vi "Config.vi"() -> ()   [LabVIEW 2020]
uses:
  Global_Variable/Global.vi
  Global_Variable/A180648.vi
  <vilib>/Utility/config.llb/NI_LVConfig.lvlib
  Libraries/S7/S7.lvlib
panel:
  in  "系数":bool
  in  "试验项目":T1
  in  "产品型号":string(combo)
  in  "删除":bool
  in  "确定":bool
  in  "添加":bool
  in  "退出":bool
  in  "更新":bool
  in  "选项卡控件":enum32{"产品参数", "系统参数"}(tab)
  in  "开启 3":string[][](table)=[["N"], ["N"], ["N"], ["mm"]]
  in  "开启 2":string[][](table)=[["N"], ["N"], ["N"], ["mm"]]
  in  "开启":string[][](table)=[["N"], ["N"], ["N"], ["mm"]]
  in  "工位坐标轴参数":string[][](table)=[["°"], ["N"], ["°"], ["N"], ["mm"], ["N"], ["mm"], ["N"]]
  in  "结果判定参数":string[][](table)=[["N"], ["N"], ["N"], ["mm"]]
  in  "系统参数设置":string[][](table)=[[""], ["mm"], ["V"], [""]]
  # "调节机构检测"
types:
  T1 = cluster{"锁紧力":bool, "开启力":bool, "推拉力":bool, "保持力":bool, "锁紧/开启":bool}
  T2 = enum8{"Enabled", "Disabled", "Disabled and Grayed Out"}
  T3 = typedef "NI_LVConfig.lvlib/Config Data RefNum.ctl" = refnum<k1>
  T4 = cluster{"[0]":cluster{string, dbl, dbl}, "[1]":cluster{string, dbl, dbl}}
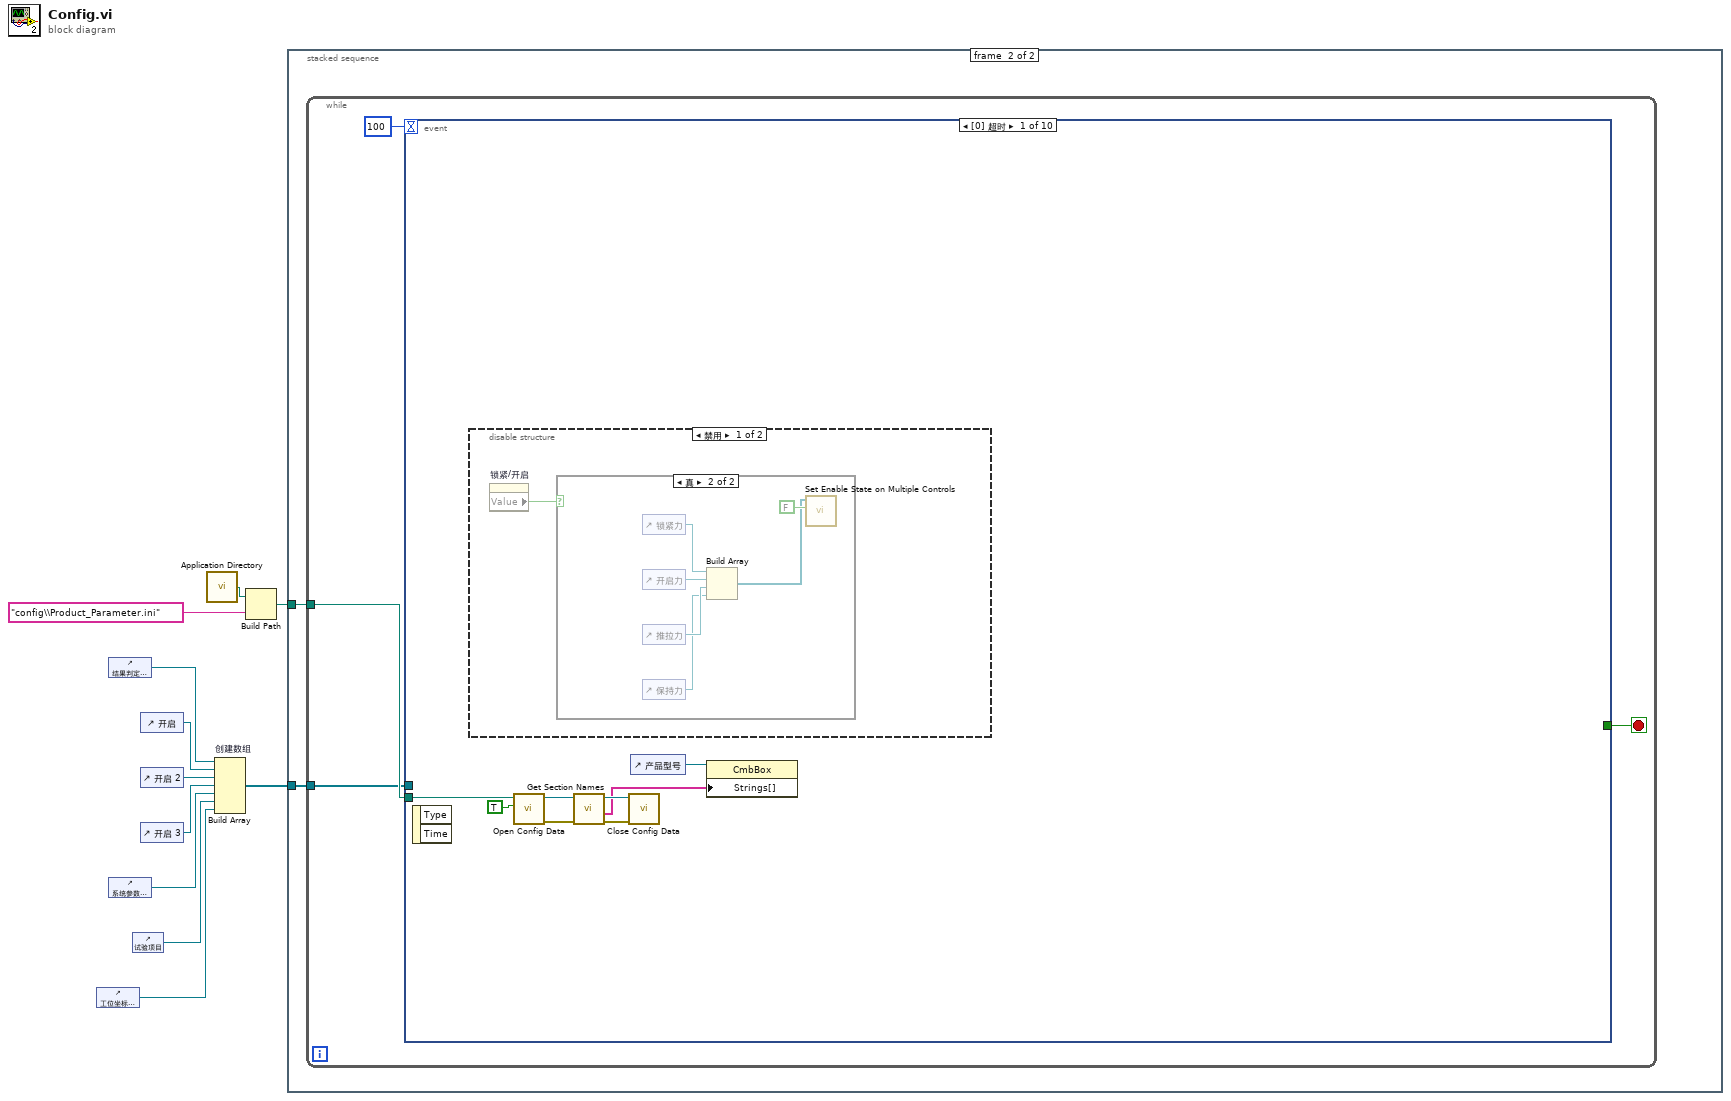
[diagram p0: block diagram]
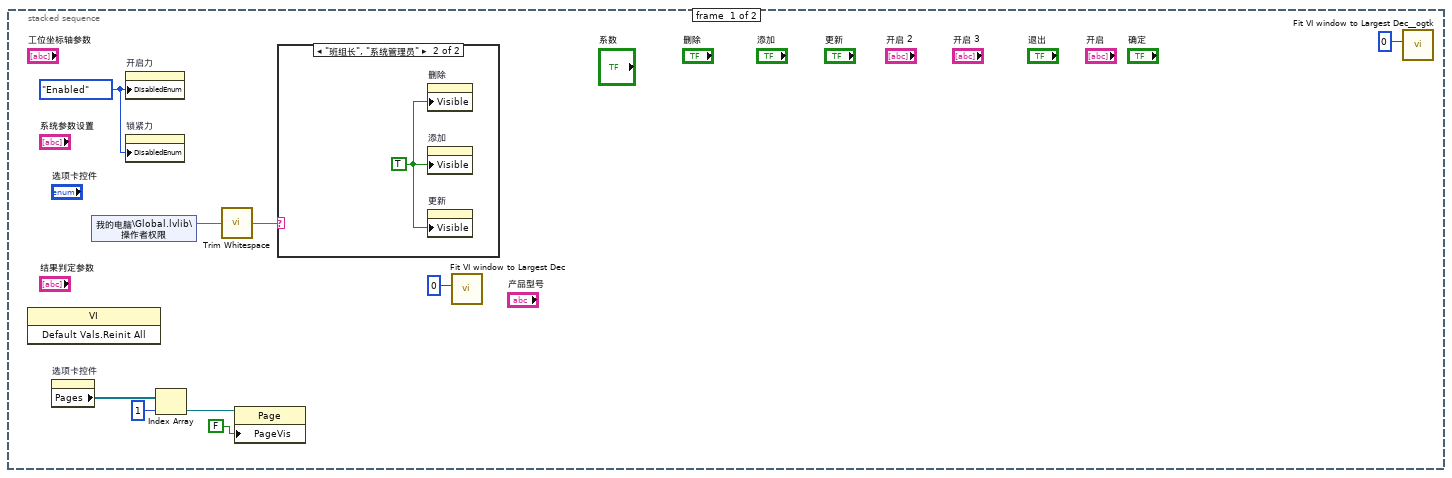
[diagram p2: hidden frame]
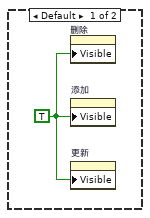
[diagram p3: hidden frame]
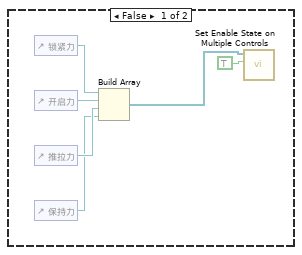
[diagram p4: hidden frame]
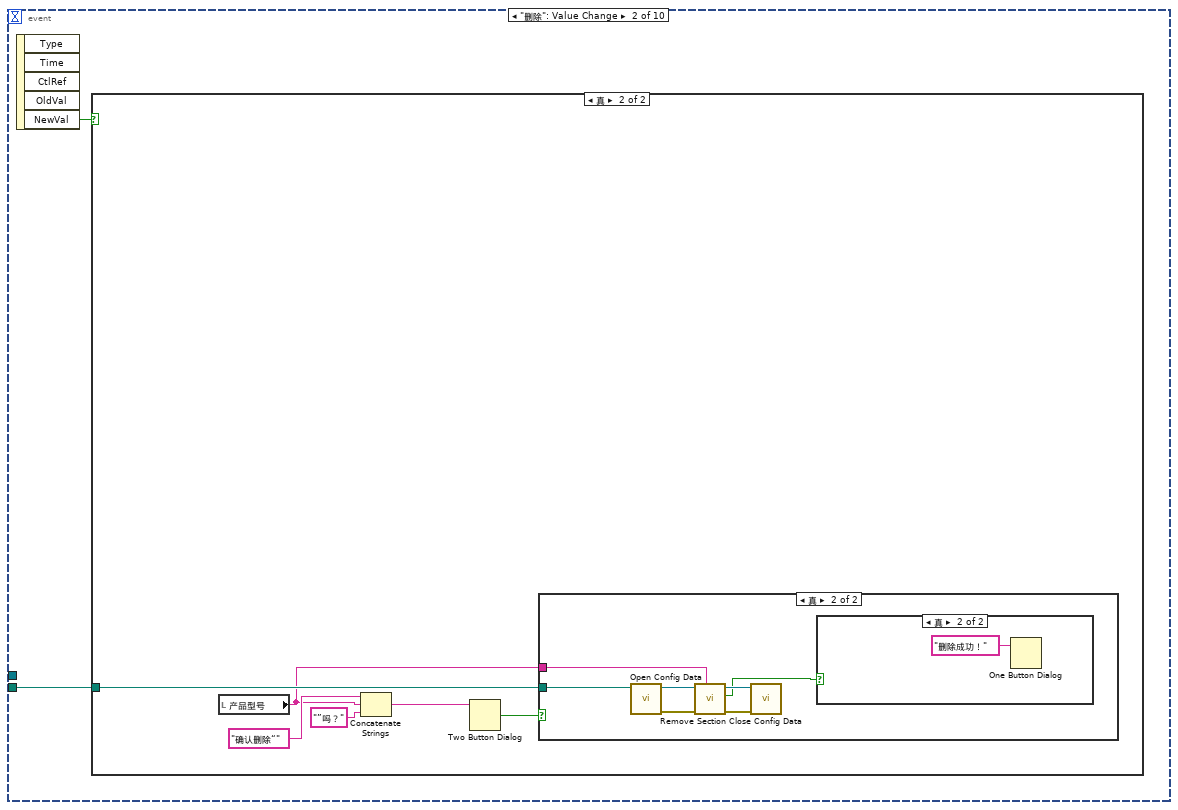
[diagram p6: hidden frame]
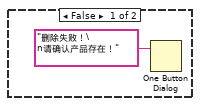
[diagram p9: hidden frame]
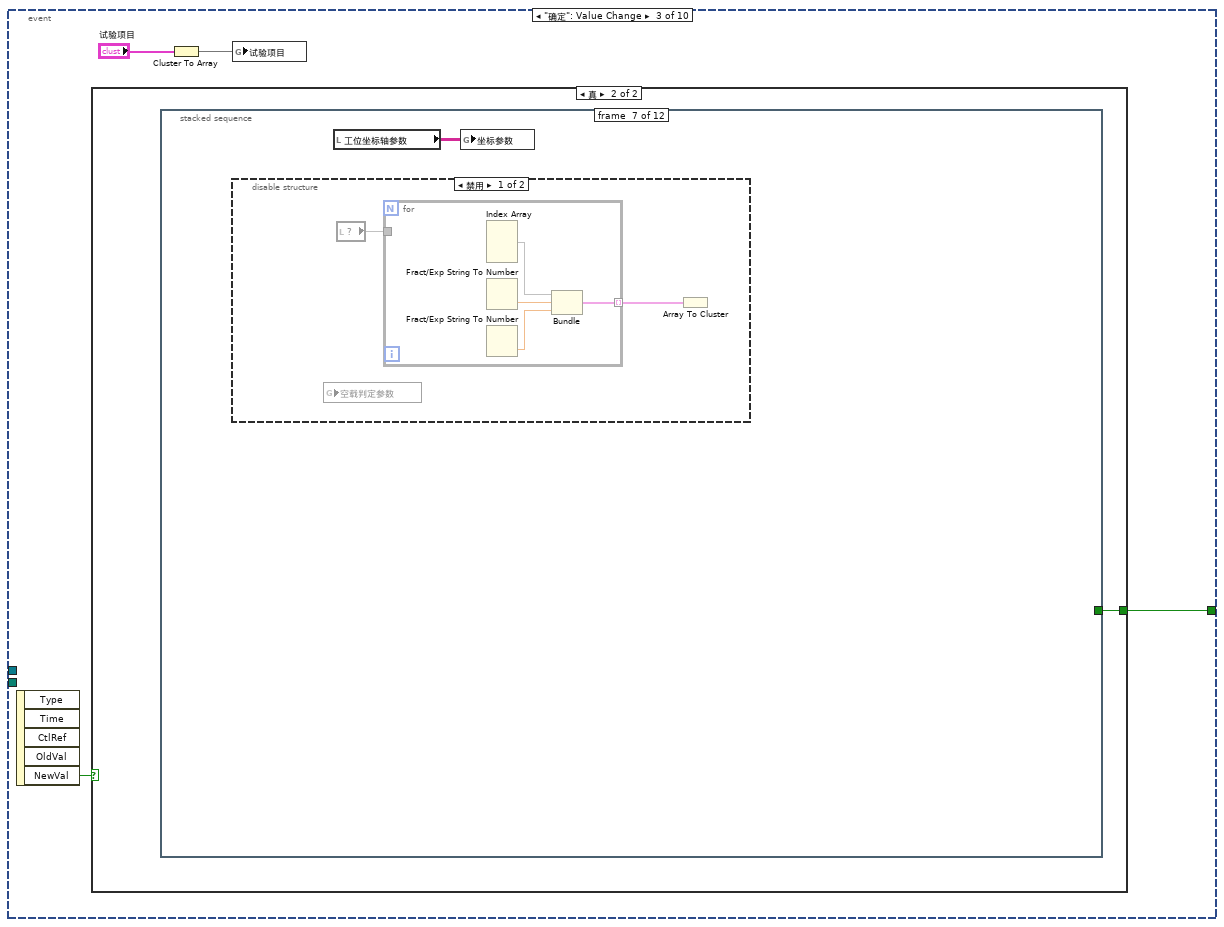
[diagram p10: hidden frame]
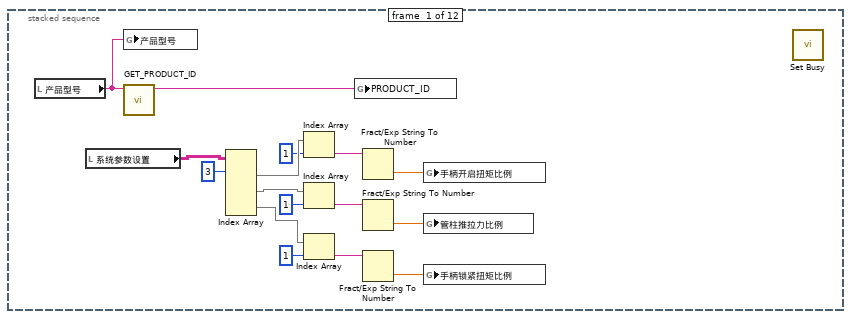
[diagram p12: hidden frame]
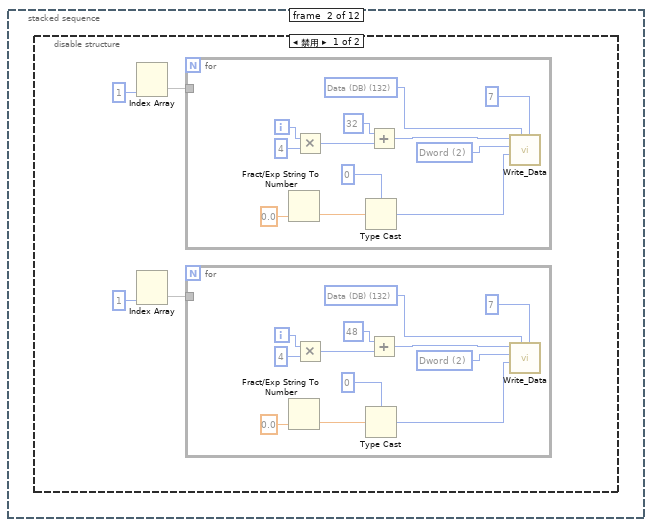
[diagram p13: hidden frame]
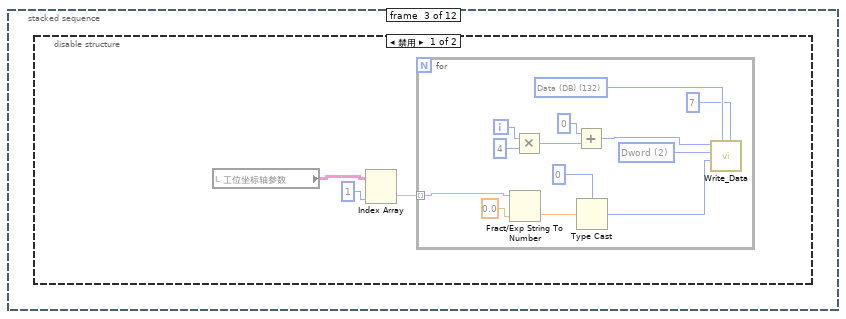
[diagram p15: hidden frame]
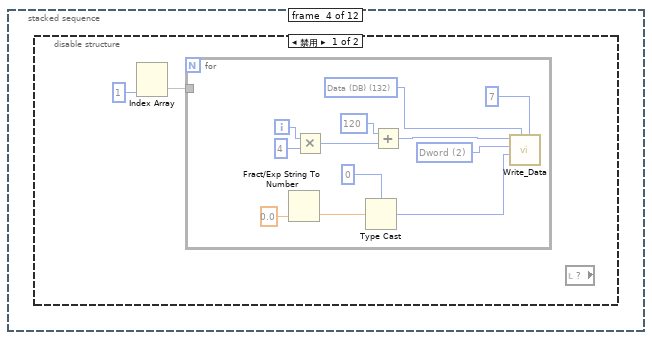
[diagram p17: hidden frame]
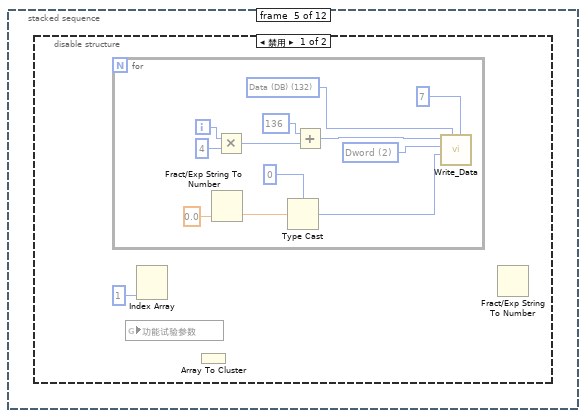
[diagram p19: hidden frame]
diagram:
  n1 = control-ref of="工位坐标轴参数"() -> (w1:refnum<vi>)
  n2 = control-ref of="结果判定参数"() -> (w7:refnum<vi>)
  n3 = control-ref of="系统参数设置"() -> (w8:refnum<vi>)
  n4 = control-ref of="试验项目"() -> (w2:refnum<vi>)
  n5 = control-ref of="开启"() -> (w5:refnum<vi>)
  n6 = control-ref of="开启 2"() -> (w4:refnum<vi>)
  n7 = control-ref of="开启 3"() -> (w3:refnum<vi>)
  n8 = call <vilib>:"Application Directory.vi"() -> ("Application Directory"=w10:path)
  n9 = Build Array "创建数组"(w7, w5, w4, w3, w8, w2, w1) -> (w11:refnum<vi>[])
  n10 = Build Path(base path=w10, name or relative path="config\\Product_Parameter.ini" ("名称或相对路径")) -> (appended path=w9:path)
  n11 = stacked-sequence {
    tunnel: w11 -> [_ w23]
    tunnel: w9 -> [_ w24]
    frame #0 {
      w16 = T2."Enabled" ("禁用")
      n12 = invoke class="VI" method="Default Vals.Reinit All"() -> ()  [unwired: 3 in, 3 out]
      n13 = property on="选项卡控件" class="TabCtl (严格)"() -> ("Pages"=w14:refnum<vi>[])  [unwired: 2 in, 2 out]
      n14 = shared-variable "我的电脑\\Global.lvlib\\操作者权限"() -> (w20:string)  [unwired: 1 in, 1 out]
      n15 = property on="开启力" class="Bool (严格)"("DisabledEnum"=w16) -> ()  [unwired: 2 in, 2 out]
      n16 = property on="锁紧力" class="Bool (严格)"("DisabledEnum"=w16) -> ()  [unwired: 2 in, 2 out]
      n17 = Index Array(array=w14, index=1 ("索引")) -> (element=w15:refnum<vi>)
      n18 = call <vilib>:"Trim Whitespace.vi"("string"=w20) -> ("trimmed string"=w19:string)  [unwired: 1 in]
      n19 = property class="Page"(reference=w15, "PageVis"=FALSE ("选项卡可见")) -> ()  [unwired: 1 in, 2 out]
      n20 = case shown="\"班组长\", \"系统管理员\"" w19 {
        frame Default {
          w21 = TRUE ("可见")
          n21 = property on="删除" class="Bool (严格)"("Visible"=w21) -> ()  [unwired: 2 in, 2 out]
          n22 = property on="添加" class="Bool (严格)"("Visible"=w21) -> ()  [unwired: 2 in, 2 out]
          n23 = property on="更新" class="Bool (严格)"("Visible"=w21) -> ()  [unwired: 2 in, 2 out]
        }
        frame "班组长", "系统管理员" {
          w22 = TRUE ("可见")
          n24 = property on="删除" class="Bool (严格)"("Visible"=w22) -> ()  [unwired: 2 in, 2 out]
          n25 = property on="添加" class="Bool (严格)"("Visible"=w22) -> ()  [unwired: 2 in, 2 out]
          n26 = property on="更新" class="Bool (严格)"("Visible"=w22) -> ()  [unwired: 2 in, 2 out]
        }
      }
      n27 = call "Fit VI window to Largest Dec.vi"("border spacing (2 px)"=0) -> ()  [unwired: 5 in, 2 out]
      n28 = call <userlib>:"Fit VI window to Largest Dec__ogtk.vi"("border spacing (2 px)"=0) -> ()  [unwired: 5 in, 2 out]
    }
    frame #1 {
      n29 = while {
        tunnel: w24 -> [w28]
        tunnel: w23 -> [w25]
        stop <- w27 stop-if-true
        n30 = event shown="[0] 超时" {
          selector: _ -> [_ _ _ _ _ _ _ _ _ _]
          dyn-events: _ -> [_ _ _ _ _ _ _ _ _ _]
          timeout: 100 -> [_ _ _ _ _ _ _ _ _ _]
          tunnel: w28 -> [w31 w51 _ w245 w273 _ w296 _ _ _]
          tunnel: [_ _ w69 _ _ TRUE _ _ _ TRUE] -> w27
          tunnel: w25 -> [_ _ _ w243 w271 _ w294 _ _ _]
          event Timeout {
            n31 = event-data() -> ()  [unwired: 1 in, 2 out]
            n32 = disable-structure shown="禁用" {
              frame Disabled {
                n33 = property on="锁紧/开启" class="Bool (严格)"() -> ("Value"=w37:bool)  [unwired: 2 in, 2 out]
                n34 = case shown="真" w37 {
                  frame False {
                    n35 = control-ref of="锁紧力"() -> (w42:refnum<vi>)
                    n36 = control-ref of="开启力"() -> (w41:refnum<vi>)
                    n37 = control-ref of="推拉力"() -> (w40:refnum<vi>)
                    n38 = control-ref of="保持力"() -> (w39:refnum<vi>)
                    n39 = Build Array(w42, w41, w40, w39) -> (w38:refnum<vi>[])
                    n40 = call "Set Enable State on Multiple Controls.vi"("启用？"=TRUE, "控件"=w38) -> ()  [unwired: 10 in]
                  }
                  frame True {
                    n41 = control-ref of="锁紧力"() -> (w48:refnum<vi>)
                    n42 = control-ref of="开启力"() -> (w47:refnum<vi>)
                    n43 = control-ref of="推拉力"() -> (w46:refnum<vi>)
                    n44 = control-ref of="保持力"() -> (w45:refnum<vi>)
                    n45 = Build Array(w48, w47, w46, w45) -> (w44:refnum<vi>[])
                    n46 = call "Set Enable State on Multiple Controls.vi"("启用？"=FALSE, "控件"=w44) -> ()  [unwired: 10 in]
                  }
                }
              }
              frame Enabled {
              }
            }
            n47 = call <vilib>:"Open Config Data.vi"("create file if necessary (T)"=TRUE, "configuration file path"=w31) -> ("error out"=w33:errorcluster, "refnum"=w32:T3)  [unwired: 7 in, 1 out]
            n48 = call <vilib>:"Get Section Names.vi"("error in (no error)"=w33, "refnum"=w32) -> ("error out"=w35:errorcluster, "section names"=w29:string[], "refnum out"=w34:T3)  [unwired: 7 in]
            n49 = call <vilib>:"Close Config Data.vi"("error in (no error)"=w35, "refnum"=w34) -> ()  [unwired: 8 in, 2 out]
            n50 = control-ref of="产品型号"() -> (w30:refnum<vi>)
            n51 = property on="属性节点" class="CmbBox"(reference=w30, "Strings[]"=w29) -> ()  [unwired: 1 in, 2 out]
          }
          event "删除": Value Change {
            n52 = event-data() -> ("NewVal"=w50:bool)  [unwired: 1 in, 4 out]
            n53 = case shown="真" w50 {
              tunnel: w51 -> [_ w53]
              frame False {
              }
              frame True {
                n54 = local read "产品型号"() -> (w52:string)
                n55 = Concatenate Strings("确认删除“", w52, "”吗？") -> (w55:string)
                n56 = Two Button Dialog(message=w55) -> (T button?=w54:bool)  [unwired: 2 in]
                n57 = case shown="真" w54 {
                  tunnel: w53 -> [_ w59]
                  tunnel: w52 -> [_ w58]
                  frame False {
                  }
                  frame True {
                    n58 = call <vilib>:"Open Config Data.vi"("configuration file path"=w59) -> ("error out"=w61:errorcluster, "refnum"=w64:T3)  [unwired: 8 in, 1 out]
                    n59 = call <vilib>:"Remove Section.vi"("section"=w58, "error in (no error)"=w61, "refnum"=w64) -> ("error out"=w63:errorcluster, "section exists?"=w60:bool, "refnum out"=w62:T3)  [unwired: 6 in]
                    n60 = call <vilib>:"Close Config Data.vi"("error in (no error)"=w63, "refnum"=w62) -> ()  [unwired: 8 in, 2 out]
                    n61 = case shown="真" w60 {
                      frame False {
                        n62 = One Button Dialog(message="删除失败！\n请确认产品存在！" ("消息")) -> ()  [unwired: 1 in, 1 out]
                      }
                      frame True {
                        n63 = One Button Dialog(message="删除成功！" ("消息")) -> ()  [unwired: 1 in, 1 out]
                      }
                    }
                  }
                }
              }
            }
          }
          event "确定": Value Change {
            n64 = event-data() -> ("NewVal"=w70:bool)  [unwired: 1 in, 4 out]
            n65 = case shown="真" w70 {
              tunnel: [_ w71] -> w69
              frame False {
              }
              frame True {
                n66 = stacked-sequence {
                  tunnel: [_ _ _ _ _ _ _ _ _ _ _ TRUE] -> w71
                  frame #0 {
                    n67 = local read "产品型号"() -> (w87:string)
                    n68 = local read "系统参数设置"() -> (w85:string[][])
                    n69 = global write "Global.vi" "产品型号"(w87) -> ()
                    n70 = call "GET_PRODUCT_ID.vi"("PRODFUCT_NAME"=w87) -> ("PRODUCT_ID"=w86:string)  [unwired: 10 in]
                    n71 = Index Array(array=w85, index (row) #1=3 ("索引 (行)")) -> (element #1=w83:string[], element #2=w77:string[], element #3=w74:string[])  [unwired: 5 in]
                    n72 = Index Array(array=w83, index=1 ("索引")) -> (element=w81:string)
                    n73 = Index Array(array=w77, index=1 ("索引")) -> (element=w79:string)
                    n74 = Index Array(array=w74, index=1 ("索引")) -> (element=w73:string)
                    n75 = global write "追溯Global.vi" "PRODUCT_ID"(w86) -> ()
                    n76 = Fract/Exp String To Number(string=w81) -> (number=w80:dbl)  [unwired: 3 in, 1 out]
                    n77 = Fract/Exp String To Number(string=w79) -> (number=w76:dbl)  [unwired: 3 in, 1 out]
                    n78 = Fract/Exp String To Number(string=w73) -> (number=w72:dbl)  [unwired: 3 in, 1 out]
                    n79 = global write "A180648.vi" "手柄开启扭矩比例"(w80) -> ()
                    n80 = global write "A180648.vi" "管柱推拉力比例"(w76) -> ()
                    n81 = global write "A180648.vi" "手柄锁紧扭矩比例"(w72) -> ()
                    n82 = call <vilib>:"Set Busy.vi"() -> ()  [unwired: 10 in, 2 out]
                  }
                  frame #1 {
                    n83 = disable-structure shown="禁用" {
                      frame Disabled {
                        n84 = Index Array(index (col)=1 ("禁用的索引 (列)")) -> (element=w91)  [unwired: 2 in]
                        n85 = Index Array(index (col)=1 ("禁用的索引 (列)")) -> (element=w88)  [unwired: 2 in]
                        n86 = for {
                          tunnel: w91 -> [_]
                          i -> [w106]
                          w113 = u16 2 items=["byte", "word", "Dword"] ("数据类型")
                          w115 = u8 132 items=["I/O (P)"=128, "Input (I)"=129, "Output (Q)"=130, "Bit Memory (M)"=131, "Data (DB)"=132, "Instance Data (DI)"=133, "Local Data (L)"=134, "Predecessor Local Data (VL)"=135] ("寄存器类型")
                          n87 = Fract/Exp String To Number(default (0 dbl)=sgl 0.0) -> (number=w110:sgl)  [unwired: 3 in, 1 out]
                          n88 = Multiply(x=w106, y=4) -> (x*y=w107:i32)
                          n89 = Type Cast(type=u32 0 ("写入地址"), x=w110) -> (*(type *) &x=w109:u32)
                          n90 = Add(x=u32 32 ("写入地址"), y=w107) -> (x+y=w104:u32)
                          n91 = call "Write_Data.vi"("DB #"=u16 7, "寄存器类型"=w115, "写入数据"=w109, "数据类型"=w113, "写入地址"=w104) -> ()  [unwired: 4 in, 3 out]
                        }
                        n92 = for {
                          tunnel: w88 -> [_]
                          i -> [w94]
                          w101 = u16 2 items=["byte", "word", "Dword"] ("数据类型")
                          w103 = u8 132 items=["I/O (P)"=128, "Input (I)"=129, "Output (Q)"=130, "Bit Memory (M)"=131, "Data (DB)"=132, "Instance Data (DI)"=133, "Local Data (L)"=134, "Predecessor Local Data (VL)"=135] ("寄存器类型")
                          n93 = Fract/Exp String To Number(default (0 dbl)=sgl 0.0) -> (number=w98:sgl)  [unwired: 3 in, 1 out]
                          n94 = Multiply(x=w94, y=4) -> (x*y=w95:i32)
                          n95 = Type Cast(type=u32 0 ("写入地址"), x=w98) -> (*(type *) &x=w97:u32)
                          n96 = Add(x=u32 48 ("写入地址"), y=w95) -> (x+y=w92:u32)
                          n97 = call "Write_Data.vi"("DB #"=u16 7, "寄存器类型"=w103, "写入数据"=w97, "数据类型"=w101, "写入地址"=w92) -> ()  [unwired: 4 in, 3 out]
                        }
                      }
                      frame Enabled {
                      }
                    }
                  }
                  frame #2 {
                    n98 = disable-structure shown="禁用" {
                      frame Disabled {
                        n99 = local read "工位坐标轴参数"() -> (w118:string[][])
                        n100 = Index Array(array=w118, index (col)=1 ("禁用的索引 (列)")) -> (element=w117:string[])  [unwired: 1 in]
                        n101 = for {
                          tunnel: w117 -> [w127] mode=indexing
                          i -> [w121]
                          w129 = u16 2 items=["byte", "word", "Dword"] ("数据类型")
                          w131 = u8 132 items=["I/O (P)"=128, "Input (I)"=129, "Output (Q)"=130, "Bit Memory (M)"=131, "Data (DB)"=132, "Instance Data (DI)"=133, "Local Data (L)"=134, "Predecessor Local Data (VL)"=135] ("寄存器类型")
                          n102 = Fract/Exp String To Number(string=w127, default (0 dbl)=sgl 0.0) -> (number=w125:sgl)  [unwired: 2 in, 1 out]
                          n103 = Multiply(x=w121, y=4) -> (x*y=w122:i32)
                          n104 = Add(x=u32 0 ("写入地址"), y=w122) -> (x+y=w119:u32)
                          n105 = Type Cast(type=u32 0 ("写入地址"), x=w125) -> (*(type *) &x=w124:u32)
                          n106 = call "Write_Data.vi"("DB #"=u16 7, "寄存器类型"=w131, "写入数据"=w124, "数据类型"=w129, "写入地址"=w119) -> ()  [unwired: 4 in, 3 out]
                        }
                      }
                      frame Enabled {
                      }
                    }
                  }
                  frame #3 {
                    n107 = disable-structure shown="禁用" {
                      frame Disabled {
                        n108 = Index Array(index (col)=1 ("禁用的索引 (列)")) -> (element=w133)  [unwired: 2 in]
                        n109 = for {
                          tunnel: w133 -> [_]
                          i -> [w136]
                          w143 = u16 2 items=["byte", "word", "Dword"] ("数据类型")
                          w145 = u8 132 items=["I/O (P)"=128, "Input (I)"=129, "Output (Q)"=130, "Bit Memory (M)"=131, "Data (DB)"=132, "Instance Data (DI)"=133, "Local Data (L)"=134, "Predecessor Local Data (VL)"=135] ("寄存器类型")
                          n110 = Fract/Exp String To Number(default (0 dbl)=sgl 0.0) -> (number=w140:sgl)  [unwired: 3 in, 1 out]
                          n111 = Multiply(x=w136, y=4) -> (x*y=w137:i32)
                          n112 = Type Cast(type=u32 0 ("写入地址"), x=w140) -> (*(type *) &x=w139:u32)
                          n113 = Add(x=u32 120 ("写入地址"), y=w137) -> (x+y=w134:u32)
                          n114 = call "Write_Data.vi"("DB #"=u16 7, "寄存器类型"=w145, "写入数据"=w139, "数据类型"=w143, "写入地址"=w134) -> ()  [unwired: 4 in, 3 out]
                        }
                        n115 = local read item#-1() -> ()  [unwired: 1 out]
                      }
                      frame Enabled {
                      }
                    }
                  }
                  frame #4 {
                    n116 = disable-structure shown="禁用" {
                      frame Disabled {
                        n117 = for {
                          i -> [w149]
                          w156 = u16 2 items=["byte", "word", "Dword"] ("数据类型")
                          w158 = u8 132 items=["I/O (P)"=128, "Input (I)"=129, "Output (Q)"=130, "Bit Memory (M)"=131, "Data (DB)"=132, "Instance Data (DI)"=133, "Local Data (L)"=134, "Predecessor Local Data (VL)"=135] ("寄存器类型")
                          n118 = Fract/Exp String To Number(default (0 dbl)=sgl 0.0) -> (number=w153:sgl)  [unwired: 3 in, 1 out]
                          n119 = Multiply(x=w149, y=4) -> (x*y=w150:i32)
                          n120 = Type Cast(type=u32 0 ("写入地址"), x=w153) -> (*(type *) &x=w152:u32)
                          n121 = Add(x=u32 136 ("写入地址"), y=w150) -> (x+y=w147:u32)
                          n122 = call "Write_Data.vi"("DB #"=u16 7, "寄存器类型"=w158, "写入数据"=w152, "数据类型"=w156, "写入地址"=w147) -> ()  [unwired: 4 in, 3 out]
                        }
                        n123 = global read "A180648.vi" "功能试验参数"() -> ()  [unwired: 1 in]
                        n124 = Index Array(index (col)=1 ("禁用的索引 (列)")) -> ()  [unwired: 2 in, 1 out]
                        n125 = Array To Cluster() -> ()  [unwired: 1 in, 1 out]
                        n126 = Fract/Exp String To Number() -> ()  [unwired: 4 in, 2 out]
                      }
                      frame Enabled {
                      }
                    }
                  }
                  frame #5 {
                    n127 = disable-structure shown="禁用" {
                      frame Disabled {
                        n128 = for {
                          i -> [w162]
                          w169 = u16 2 items=["byte", "word", "Dword"] ("数据类型")
                          w171 = u8 132 items=["I/O (P)"=128, "Input (I)"=129, "Output (Q)"=130, "Bit Memory (M)"=131, "Data (DB)"=132, "Instance Data (DI)"=133, "Local Data (L)"=134, "Predecessor Local Data (VL)"=135] ("寄存器类型")
                          n129 = Fract/Exp String To Number(default (0 dbl)=sgl 0.0) -> (number=w166:sgl)  [unwired: 3 in, 1 out]
                          n130 = Multiply(x=w162, y=4) -> (x*y=w163:i32)
                          n131 = Type Cast(type=u32 0 ("写入地址"), x=w166) -> (*(type *) &x=w165:u32)
                          n132 = Add(x=u32 168 ("写入地址"), y=w163) -> (x+y=w160:u32)
                          n133 = call "Write_Data.vi"("DB #"=u16 7, "寄存器类型"=w171, "写入数据"=w165, "数据类型"=w169, "写入地址"=w160) -> ()  [unwired: 4 in, 3 out]
                        }
                        n134 = global read "A180648.vi" "逆向空载试验参数"() -> ()  [unwired: 1 in]
                        n135 = Index Array(index (col)=1 ("禁用的索引 (列)")) -> ()  [unwired: 2 in, 1 out]
                        n136 = Fract/Exp String To Number() -> ()  [unwired: 4 in, 2 out]
                        n137 = Array To Cluster() -> ()  [unwired: 1 in, 1 out]
                      }
                      frame Enabled {
                      }
                    }
                  }
                  frame #6 {
                    n138 = disable-structure shown="禁用" {
                      frame Disabled {
                        n139 = global read "判定参数.vi" "空载判定参数"() -> ()  [unwired: 1 in]
                        n140 = local read item#-1() -> (w174)
                        n141 = for {
                          tunnel: w174 -> [_]
                          tunnel: [w176] -> w173 mode=indexing
                          n142 = Index Array() -> (element #1=w175)  [unwired: 4 in, 2 out]
                          n143 = Fract/Exp String To Number() -> (number=w178:dbl)  [unwired: 4 in, 1 out]
                          n144 = Fract/Exp String To Number() -> (number=w177:dbl)  [unwired: 4 in, 1 out]
                          n145 = Bundle(w175, w178, w177) -> (w176:cluster{void, dbl, dbl})  [unwired: 1 in]
                        }
                        n146 = Array To Cluster(array=w173) -> ()  [unwired: 1 out]
                      }
                      frame Enabled {
                      }
                    }
                    n147 = local read "工位坐标轴参数"() -> (w172:string[][])
                    n148 = global write "A180648.vi" "坐标参数"(w172) -> ()
                  }
                  frame #7 {
                    w179 = 1 ("索引")
                    n149 = local read "开启 3"() -> (w192:string[][])
                    n150 = local read "开启 2"() -> (w196:string[][])
                    n151 = local read "开启"() -> (w199:string[][])
                    n152 = for {
                      tunnel: w199 -> [w223] mode=indexing
                      tunnel: [w225] -> w198 mode=indexing
                      n153 = Index Array(array=w223, index #1=0) -> (element #1=w224:string, element #2=w222:string, element #3=w221:string)  [unwired: 2 in]
                      n154 = Fract/Exp String To Number(string=w222) -> (number=w227:dbl)  [unwired: 3 in, 1 out]
                      n155 = Fract/Exp String To Number(string=w221) -> (number=w226:dbl)  [unwired: 3 in, 1 out]
                      n156 = Bundle(w224, w227, w226) -> (w225:cluster{string, dbl, dbl})  [unwired: 1 in]
                    }
                    n157 = for {
                      tunnel: w192 -> [w208] mode=indexing
                      tunnel: [w204] -> w194 mode=indexing
                      n158 = Index Array(array=w208, index #1=0) -> (element #1=w209:string, element #2=w207:string, element #3=w206:string)  [unwired: 2 in]
                      n159 = Fract/Exp String To Number(string=w207) -> (number=w211:dbl)  [unwired: 3 in, 1 out]
                      n160 = Fract/Exp String To Number(string=w206) -> (number=w210:dbl)  [unwired: 3 in, 1 out]
                      n161 = Bundle(w209, w211, w210) -> (w204:cluster{string, dbl, dbl})  [unwired: 1 in]
                    }
                    n162 = for {
                      tunnel: w196 -> [w215] mode=indexing
                      tunnel: [w217] -> w195 mode=indexing
                      n163 = Index Array(array=w215, index #1=0) -> (element #1=w216:string, element #2=w214:string, element #3=w213:string)  [unwired: 2 in]
                      n164 = Fract/Exp String To Number(string=w214) -> (number=w219:dbl)  [unwired: 3 in, 1 out]
                      n165 = Fract/Exp String To Number(string=w213) -> (number=w218:dbl)  [unwired: 3 in, 1 out]
                      n166 = Bundle(w216, w219, w218) -> (w217:cluster{string, dbl, dbl})  [unwired: 1 in]
                    }
                    n167 = Index Array(array=w192, index (row) #1=1 ("索引 (行)"), index (row) #2=2 ("索引 (行)")) -> (element #1=w190:string[], element #2=w185:string[])  [unwired: 4 in, 1 out]
                    n168 = local read "结果判定参数"() -> (w202:string[][])
                    n169 = Index Array(array=w190, index #1=w179) -> (element #1=w189:string, element #2=w187:string)  [unwired: 1 in]
                    n170 = Index Array(array=w185, index #1=w179) -> (element #1=w184:string, element #2=w183:string)  [unwired: 1 in]
                    n171 = for {
                      tunnel: w202 -> [w231] mode=indexing
                      tunnel: [w233] -> w203 mode=indexing
                      n172 = Index Array(array=w231, index #1=0) -> (element #1=w232:string, element #2=w230:string, element #3=w229:string)  [unwired: 2 in]
                      n173 = Fract/Exp String To Number(string=w230) -> (number=w235:dbl)  [unwired: 3 in, 1 out]
                      n174 = Fract/Exp String To Number(string=w229) -> (number=w234:dbl)  [unwired: 3 in, 1 out]
                      n175 = Bundle(w232, w235, w234) -> (w233:cluster{string, dbl, dbl})  [unwired: 1 in]
                    }
                    n176 = Fract/Exp String To Number(string=w183) -> (number=w181:dbl)  [unwired: 3 in, 1 out]
                    n177 = Fract/Exp String To Number(string=w189) -> (number=w188:dbl)  [unwired: 3 in, 1 out]
                    n178 = Fract/Exp String To Number(string=w187) -> (number=w186:dbl)  [unwired: 3 in, 1 out]
                    n179 = Fract/Exp String To Number(string=w184) -> (number=w182:dbl)  [unwired: 3 in, 1 out]
                    n180 = global write "判定参数.vi" "最大拉力"(w181) -> ()
                    n181 = global write "判定参数.vi" "最小位移"(w188) -> ()
                    n182 = global write "判定参数.vi" "最大位移"(w186) -> ()
                    n183 = global write "判定参数.vi" "最小拉力"(w182) -> ()
                    n184 = Array To Cluster(array=w198) -> (cluster=w200:cluster{"[0]":cluster{string, dbl, dbl}})
                    n185 = Array To Cluster(array=w194) -> (cluster=w193:T4)
                    n186 = Array To Cluster(array=w195) -> (cluster=w197:cluster{"[0]":cluster{string, dbl, dbl}})
                    n187 = global write "判定参数.vi" "开启判定参数"(w200) -> ()
                    n188 = global write "判定参数.vi" "保持力判定参数"(w193) -> ()
                    n189 = global write "判定参数.vi" "推拉力判定参数"(w197) -> ()
                    n190 = Array To Cluster(array=w203) -> (cluster=w201:cluster{"[0]":cluster{string, dbl, dbl}})
                    n191 = global write "判定参数.vi" "锁紧判定参数"(w201) -> ()
                  }
                  frame #8 {
                    n192 = call <vilib>:"Unset Busy.vi"() -> ()  [unwired: 11 in, 1 out]
                  }
                  frame #9 {
                    n193 = global read "Global.vi" "更换产品"() -> (w237:refnum<vi>)
                    n194 = global read "Global.vi" "更换坐标"() -> (w239:refnum<vi>)
                    n195 = vi-ref "Main.vi"() -> (w236:refnum<vi>)
                    n196 = vi-ref "Auto.vi"() -> (w238:refnum<vi>)
                    n197 = property class="VIRef"(reference=w237, "Val(Sgnl)"=w236) -> ()  [unwired: 1 in, 2 out]
                    n198 = property class="VIRef"(reference=w239, "Val(Sgnl)"=w238) -> ()  [unwired: 1 in, 2 out]
                  }
                  frame #10 {
                    w240 = "参数装载成功！" ("消息")
                    n199 = call "浮动通知.vi"("通知内容"=w240) -> ()  [unwired: 11 in]
                    n200 = One Button Dialog(message=w240) -> ()  [unwired: 1 in, 1 out]
                  }
                  frame #11 {
                    n201 = control-ref of="本VI"() -> (w241:refnum<vi>)
                    n202 = invoke class="VI" method="FP.Close"(reference=w241) -> ()  [unwired: 2 in, 3 out]
                  }
                }
              }
            }
            n203 = Cluster To Array(cluster="试验项目") -> (array=w67:bool[])
            n204 = global write "Global.vi" "试验项目"(w67) -> ()
          }
          event "添加": Value Change {
            n205 = event-data() -> ("NewVal"=w244:bool)  [unwired: 1 in, 4 out]
            n206 = case shown="真" w244 {
              tunnel: w245 -> [_ w249]
              tunnel: w243 -> [_ w246]
              frame False {
              }
              frame True {
                n207 = call "产品添加提示：用户输入"() -> ("产品型号"=w247:string, "确定"=w248:bool)  [unwired: 17 in, 1 out]
                n208 = case shown="真" w248 {
                  tunnel: w249 -> [_ w252]
                  tunnel: w247 -> [_ w251]
                  tunnel: w246 -> [_ w250]
                  frame False {
                  }
                  frame True {
                    n209 = case shown="默认" w251 {
                      selector: w251 -> [_ w256]
                      tunnel: w252 -> [_ w258]
                      tunnel: w250 -> [_ w254]
                      frame "" {
                        n210 = One Button Dialog(message="产品名称不得为空!" ("text")) -> ()  [unwired: 1 in, 1 out]
                      }
                      frame Default {
                        n211 = property on="产品型号" class="CmbBox"() -> ("Strings[]"=w257:string[])  [unwired: 2 in, 2 out]
                        n212 = Search 1D Array(1D array=w257, element=w256) -> (index of element=w255:i32)  [unwired: 1 in]
                        n213 = case shown="-1" w255 {
                          tunnel: w258 -> [_ w262]
                          tunnel: w256 -> [_ w261]
                          tunnel: w254 -> [_ w260]
                          frame Default {
                            n214 = One Button Dialog(message="产品已存在！" ("消息")) -> ()  [unwired: 1 in, 1 out]
                          }
                          frame -1 {
                            n215 = stacked-sequence {
                              tunnel: w262 -> [w265 _]
                              tunnel: w261 -> [w264 _]
                              tunnel: w260 -> [w263 _]
                              frame #0 {
                                n216 = for {
                                tunnel: w265 -> [w269]
                                tunnel: w264 -> [w266]
                                tunnel: w263 -> [w268] mode=indexing
                                n217 = control-ref of="工位坐标轴参数"() -> ()  [unwired: 1 out]
                                n218 = call "Read_Write ParaINI File.vi"("Mode"=enum16{"Read", "Write"}."Write", "Section"=w266, "Filepath"=w269, "Ctl Refnum"=w268) -> ()  [unwired: 7 in, 1 out]
                                }
                              }
                              frame #1 {
                                n219 = One Button Dialog(message="添加成功！" ("消息")) -> ()  [unwired: 1 in, 1 out]
                              }
                            }
                          }
                        }
                      }
                    }
                  }
                }
              }
            }
          }
          event "产品型号": Value Change {
            n220 = event-data() -> ("NewVal"=w272:string)  [unwired: 1 in, 4 out]
            n221 = stacked-sequence {
              tunnel: w273 -> [_ _ w277]
              tunnel: w272 -> [_ w275 _]
              tunnel: w271 -> [_ _ w276]
              frame #0 {
                n222 = control-ref of="本VI"() -> (w274:refnum<vi>)
                n223 = invoke class="VI" method="Default Vals.Reinit All"(reference=w274) -> ()  [unwired: 2 in, 3 out]
              }
              frame #1 {
                n224 = local write "产品型号"(w275) -> ()
              }
              frame #2 {
                n225 = disable-structure shown="启用" {
                  disable-tunnel: w277 -> [w278 w286]
                  disable-tunnel: w276 -> [_ w287]
                  frame Disabled {
                    n226 = for {
                      tunnel: [w282] -> w279 mode=indexing
                      tunnel: w278 -> [w281]
                      n227 = local read "产品型号"() -> (w280:string)
                      n228 = call "Read_Write ParaINI File.vi"("Mode"=enum16{"Read", "Write"}."Read", "Section"=w280, "Filepath"=w281, "Ctl Refnum"=w282) -> ()  [unwired: 7 in, 1 out]
                    }
                  }
                  frame Enabled {
                    n229 = local read "产品型号"() -> (w288:string)
                    n230 = call <vilib>:"Set Busy.vi"() -> ("error out"=w285:errorcluster)  [unwired: 10 in, 1 out]
                    n231 = call "Read_Write INI File.vi"("Mode"=enum16{"Read", "Write"}."Read", "Section"=w288, "error in"=w285, "Filepath"=w286, "Ctl Refnum"=w287) -> ("error out"=w284:errorcluster)  [unwired: 6 in]
                    n232 = call <vilib>:"Unset Busy.vi"("error in (no error)"=w284) -> ()  [unwired: 10 in, 1 out]
                  }
                }
              }
            }
          }
          event "退出": Value Change {
            n233 = event-data() -> ()  [unwired: 1 in, 5 out]
            n234 = control-ref of="本VI"() -> (w292:refnum<vi>)
            n235 = invoke class="VI" method="FP.Close"(reference=w292) -> (reference out=w290:refnum<vi>, error out=w291:errorcluster)  [unwired: 2 in, 1 out]
            n236 = Close Reference(reference=w290, error in (no error)=w291) -> ()  [unwired: 1 out]
          }
          event "更新": Value Change {
            n237 = event-data() -> ("NewVal"=w295:bool)  [unwired: 1 in, 4 out]
            n238 = case shown="真" w295 {
              tunnel: w296 -> [_ w299]
              tunnel: w294 -> [_ w297]
              frame False {
              }
              frame True {
                n239 = for {
                  tunnel: w299 -> [w306]
                  tunnel: [w305] -> w298
                  tunnel: w297 -> [w304] mode=indexing
                  n240 = local read "产品型号"() -> (w308:string)
                  n241 = call "Read_Write ParaINI File.vi"("Mode"=enum16{"Read", "Write"}."Write", "Section"=w308, "Filepath"=w306, "Ctl Refnum"=w304) -> ("error out"=w305:errorcluster)  [unwired: 7 in]
                }
                n242 = case shown="无错误" w298 {
                  frame No Error {
                    n243 = Wait (ms)(milliseconds to wait=u32 500 ("等待时间（毫秒）")) -> ()  [unwired: 1 out]
                    n244 = One Button Dialog(message="更新成功！" ("通知内容")) -> ()  [unwired: 1 in, 1 out]
                  }
                  frame Error {
                    n245 = Wait (ms)(milliseconds to wait=u32 500 ("等待时间（毫秒）")) -> ()  [unwired: 1 out]
                    n246 = call "浮动通知.vi"("通知内容"="更新失败！") -> ()  [unwired: 11 in]
                  }
                }
              }
            }
          }
          event "系数": Mouse Enter {
            n247 = event-data() -> ()  [unwired: 1 in, 4 out]
            n248 = property on="系数" class="Bool"("Colors [4]"=cluster{u32, u32}[] [{16777216, 16777216}] ("颜色[4]")) -> ()  [unwired: 2 in, 2 out]
          }
          event "系数": Value Change {
            n249 = event-data() -> ("NewVal"=w311:bool)  [unwired: 1 in, 5 out]
            n250 = property on="选项卡控件" class="TabCtl (严格)"() -> ("Pages"=w313:refnum<vi>[])  [unwired: 2 in, 2 out]
            n251 = Index Array(array=w313, index=1 ("索引")) -> (element=w312:refnum<vi>)
            n252 = property class="Page"(reference=w312, "PageVis"=w311) -> ()  [unwired: 1 in, 2 out]
          }
          event Panel Close {
            n253 = event-data() -> ()  [unwired: 1 in, 3 out]
          }
        }
      }
    }
  }
